vi "Open vi Reference_2.1.0.0.vi"(4 "Close Front Panel(T)":bool, 5 "Wait Until Done":bool=TRUE, 6 "Front Panel State":T1(ring)=enum."Standard", 7 "Auto Dispose Reference":bool, 8 "error in":errorcluster, 10 "vi path":path) -> (0 "error out":errorcluster, 2 "vi reference":refnum<vi>, 3 "History:Revision Number":string)   [LabVIEW 2018]
uses:
  <vilib>/Utility/error.llb/DialogType.ctl
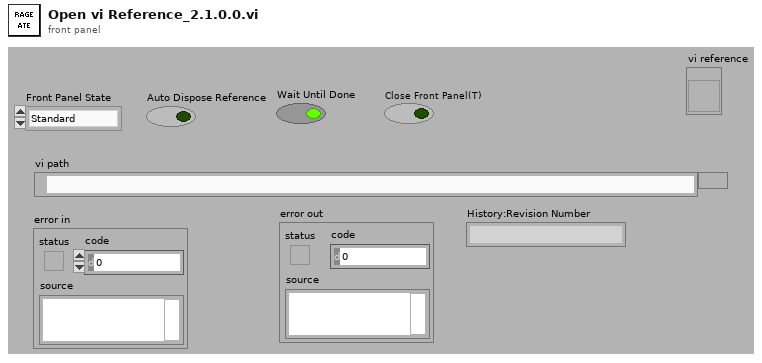
[diagram p1: front panel]
types:
  T1 = enum32{"Invalid", "Standard", "Closed", "Hidden", "Minimized", "Maximized"}
  T2 = typedef "DialogType.ctl" = u16
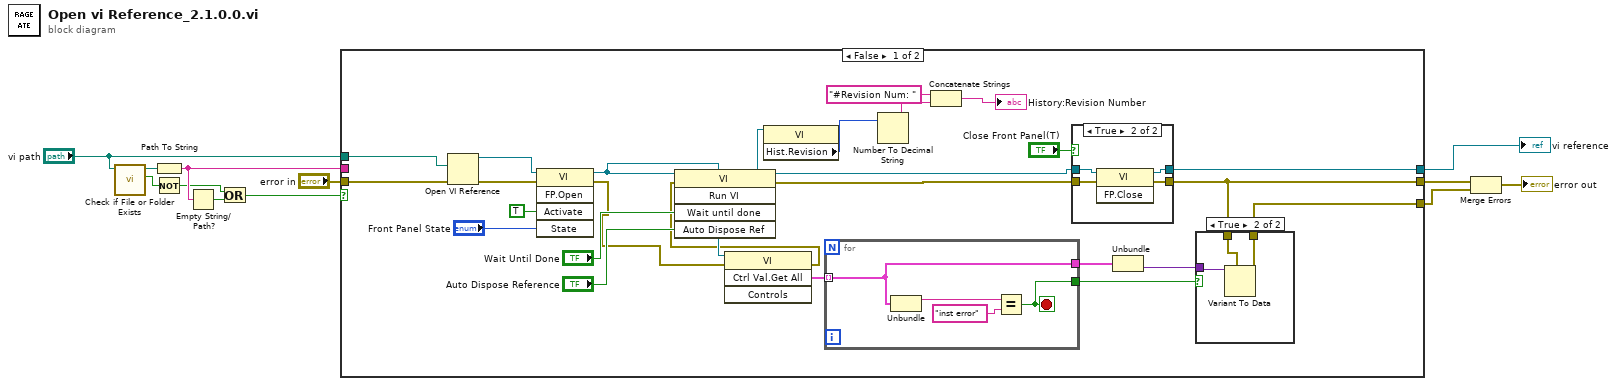
[diagram p0: block diagram]
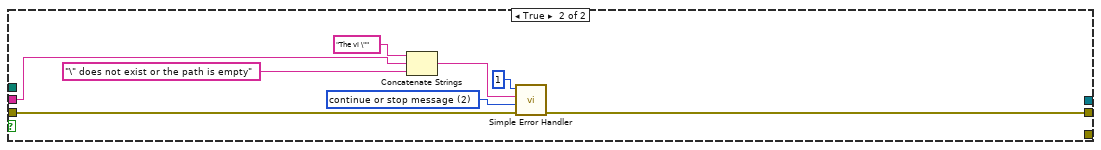
[diagram p4: hidden frame]
diagram:
  n1 = call <vilib>:"Check if File or Folder Exists.vi"("path"="vi path") -> ("file or folder exists?"=w7:bool, "dup path"=w9:path)  [unwired: 8 in, 1 out]
  n2 = Path To String(path=w9) -> (string=w8:string)
  n3 = Not(x=w7) -> (.not. x?=w4:bool)
  n4 = Empty String/Path?(string/path=w8) -> (empty?=w5:bool)
  n5 = Or(x=w4, y=w5) -> (x .or. y?=w6:bool)
  n6 = case shown="False" w6 {
    tunnel: [w37 _] -> w12
    tunnel: "vi path" -> [w35 _]
    tunnel: "error in" -> [w28 w58]
    tunnel: [w25 w52] -> w3
    tunnel: w8 -> [_ w53]
    tunnel: [w24 _] -> w1
    frame False {
      n7 = Open VI Reference(vi path=w35, error in (no error)=w28) -> (vi reference=w29:refnum<vi>, error out=w32:errorcluster)  [unwired: 4 in]
      n8 = invoke class="VI" method="FP.Open"(reference=w29, error in=w32, "Activate"=TRUE ("Activate FP?"), "State"="Front Panel State") -> (reference out=w15:refnum<vi>, error out=w14:errorcluster)  [unwired: 1 in, 3 out]
      n9 = invoke class="VI" method="Ctrl Val.Get All"(reference=w15, error in=w14) -> (error out=w13:errorcluster, "Get All Control Values Variant"=w23:cluster{"Name":string, "Variant Data":variant}[])  [unwired: 2 in, 2 out]
      n10 = invoke class="VI" method="Run VI"(reference=w15, error in=w13, "Wait until done"="Wait Until Done", "Auto Dispose Ref"="Auto Dispose Reference") -> (reference out=w20:refnum<vi>, error out=w36:errorcluster)  [unwired: 1 in, 3 out]
      n11 = property class="VI"(reference=w20) -> ("Hist.Revision"=w19:u32)  [unwired: 1 in, 2 out]
      n12 = for {
        tunnel: w23 -> [w43] mode=indexing
        tunnel: [w43] -> w22
        tunnel: [w42] -> w21
        stop <- w42 stop-if-true
        n13 = Unbundle(w43) -> ("Name"=w45:string)  [unwired: 1 out]
        n14 = Equal?(x=w45, y="inst error") -> (x = y?=w42:bool)
      }
      n15 = Number To Decimal String(number=w19) -> (decimal integer string=w18:string)  [unwired: 1 in]
      n16 = Concatenate Strings("#Revision Num: " ("string"), w18) -> (→"History:Revision Number":string)
      n17 = case shown="True" "Close Front Panel(T)" {
        tunnel: [w47 w51] -> w37
        tunnel: w36 -> [w46 w50]
        tunnel: w20 -> [w47 w49]
        tunnel: [w46 w48] -> w25
        frame False {
        }
        frame True {
          n18 = invoke class="VI" method="FP.Close"(reference=w49, error in=w50) -> (reference out=w51:refnum<vi>, error out=w48:errorcluster)  [unwired: 1 in, 1 out]
        }
      }
      n19 = Unbundle(w22) -> ("Variant Data"=w26:variant)  [unwired: 1 out]
      n20 = case shown="True" w21 {
        tunnel: w26 -> [_ w41]
        tunnel: w25 -> [w38 w40]
        tunnel: [w38 w39] -> w24
        frame False {
        }
        frame True {
          n21 = Variant To Data(type=w40, Variant=w41) -> (data=w39:errorcluster)  [unwired: 1 in, 1 out]
        }
      }
    }
    frame True {
      w59 = T2 2 items=["no dialog", "OK message", "continue or stop message", "OK message + warnings", "continue/stop + warnings"] ("type of dialog (OK msg:1)")
      n22 = Concatenate Strings("The vi \"", w53, "\" does not exist or the path is empty" ("string")) -> (w56:string)
      n23 = call <vilib>:"Simple Error Handler.vi"("error code (no error:0)"=1, "error source (\" \")"=w56, "type of dialog (OK msg:1)"=w59, "error in (no error)"=w58) -> ("error out"=w52:errorcluster)  [unwired: 1 in, 4 out]
    }
  }
  "vi reference" <- w12
  n24 = Merge Errors(w3, w1) -> (→"error out":errorcluster)
